vi "Change Scroll Position.vi"(8 "error in (no error)":errorcluster, 10 "Position Change":i32, 11 "ScrollingList in":refnum<class "ScrollingList.lvclass">) -> (0 "error out":errorcluster, 3 "ScrollingList out":refnum<class "ScrollingList.lvclass">)   [LabVIEW 2020, in "ScrollingList.lvclass"]
uses:
  ScrollingList.lvclass
  C:/Program Files/National Instruments/LabVIEW 2020/vi.lib/QSI/QControls/QControl Classes/Picture/Picture.lvclass
  ScrollingList.lvclass/ScrollingList.ctl
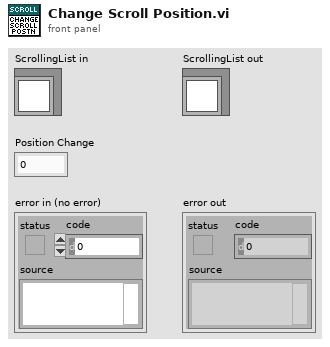
[diagram p1: front panel]
types:
  T1 = typedef "ScrollingList.lvclass/State Data.ctl" = cluster{"Timeout":i32, "Time":timestamp, "Y":i32, "Origin:Top":i16, "Rate":dbl, "ListItems":string[], "Item Height":i32, "Max Height":i32}
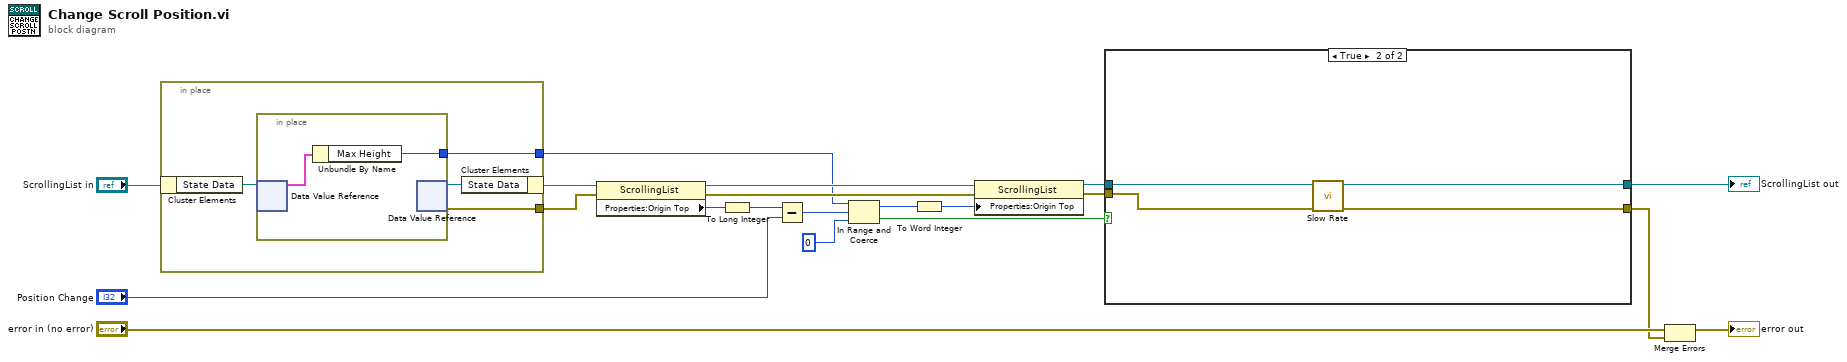
[diagram p0: block diagram]
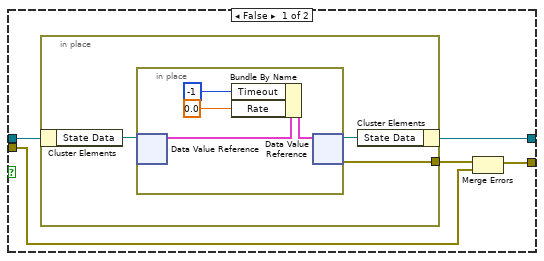
[diagram p2: hidden frame]
diagram:
  n1 = in-place {
    in-place-border: [w22] -> w8
    in-place-border: [w21] -> w10
    n2 = in-place-cluster #1("ScrollingList in") -> ("State Data"=w24:refnum<data-value>)
    n3 = in-place {
      in-place-border: [w25] -> w22
      n4 = in-place-dvr #2(w24) -> (w26:T1)  [unwired: 1 out]
      n5 = Unbundle By Name(w26) -> ("Max Height"=w25:i32)
      n6 = in-place-dvr #2() -> (w23:refnum<data-value>, w21:errorcluster)  [unwired: 1 in]
    }
    n7 = in-place-cluster #1("State Data"=w23) -> (w12:refnum<class "ScrollingList.lvclass">)
  }
  n8 = property on="Property Node" class="ScrollingList"(reference=w12, error in=w10) -> (reference out=w16:refnum<class "ScrollingList.lvclass">, error out=w9:errorcluster, "Properties:Origin Top"=w15:i16)
  n9 = To Long Integer(number=w15) -> (32bit integer=w17:i32)
  n10 = Subtract(x=w17, y="Position Change") -> (x-y=w18:i32)
  n11 = In Range and Coerce(upper limit=w8, x=w18, lower limit=0) -> (coerced(x)=w19:i32, In Range?=w7:bool)
  n12 = To Word Integer(number=w19) -> (16bit integer=w13:i16)
  n13 = property on="Property Node" class="ScrollingList"(reference=w16, error in=w9, "Properties:Origin Top"=w13) -> (reference out=w6:refnum<class "ScrollingList.lvclass">, error out=w4:errorcluster)
  n14 = case shown="True" w7 {
    tunnel: w6 -> [w31 w42]
    tunnel: [w30 w41] -> w5
    tunnel: w4 -> [w27 w40]
    tunnel: [w28 w39] -> w1
    frame False {
      n15 = in-place {
        in-place-border: [w32] -> w29
        n16 = in-place-cluster #3(w31) -> ("State Data"=w34:refnum<data-value>)
        n17 = in-place {
          n18 = in-place-dvr #4(w34) -> (w36:T1)  [unwired: 1 out]
          n19 = Bundle By Name(cluster=w36, "Timeout"=-1, "Rate"=0.0) -> (w35:T1)
          n20 = in-place-dvr #4(w35) -> (w33:refnum<data-value>, w32:errorcluster)
        }
        n21 = in-place-cluster #3("State Data"=w33) -> (w30:refnum<class "ScrollingList.lvclass">)
      }
      n22 = Merge Errors(w29, w27) -> (w28:errorcluster)
    }
    frame True {
      n23 = call "Slow Rate.vi"("error in (no error)"=w40, "ScrollingList in"=w42) -> ("error out"=w39:errorcluster, "ScrollingList out"=w41:refnum<class "ScrollingList.lvclass">)  [unwired: 8 in]
    }
  }
  "ScrollingList out" <- w5
  n24 = Merge Errors("error in (no error)", w1) -> (→"error out":errorcluster)
